vi "Encoder Get To Set Point.vi"(0 "refnum name":string="My Encoder RefNum", 1 "X":dbl, 2 "Y":dbl, 3 "setpoint":dbl format="%.2f", 4 "Enable?":bool) -> (5 "Enable?":bool, 6 "X out":dbl, 7 "Y out":dbl)   [LabVIEW 2016]
doc: "Get to a specific encoder distance (m)."
uses:
  <vilib>/addons/control/pid/pid.llb/PID (DBL).vi
  <vilib>/addons/control/pid/NI_PID_pid.lvlib
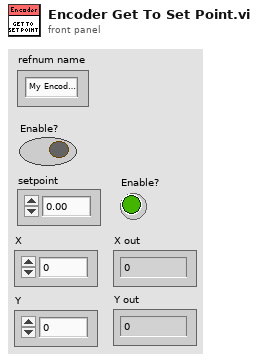
[diagram p1: front panel]
types:
  T1 = cluster{"proportional gain (Kc)":dbl, "integral time (Ti, min)":dbl, "derivative time (Td, min)":dbl}
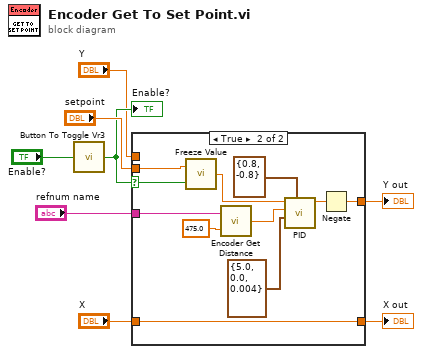
[diagram p0: block diagram]
diagram:
  n1 = call "Button To Toggle Vr3.vi"("InValue"="Enable?") -> ("Result"=w5:bool)
  "Enable?" <- w5
  n2 = case shown="True" w5 {
    selector: w5 -> [_ w12]
    tunnel: "setpoint" -> [_ w14]
    tunnel: "refnum name" -> [_ w18]
    tunnel: [w10 w15] -> w1
    tunnel: [w9 w16] -> w4
    tunnel: "X" -> [w9 w16]
    tunnel: "Y" -> [w10 _]
    frame False {
    }
    frame True {
      n3 = call "Freeze Value.vi"("Freeze Value"=w12, "In Value"=w14) -> ("Value Out"=w13:dbl)
      n4 = call "Encoder Get Distance.vi"("Distance/Meter ratio"=475.0, "refnum name"=w18) -> ("Distance (m)"=w20:dbl)
      n5 = call-poly <vilib>:"PID.vi"("output range"=cluster{"output high":dbl, "output low":dbl} {"output high"=0.8, "output low"=-0.8}, "PID gains"=T1 {"proportional gain (Kc)"=5.0, "integral time (Ti, min)"=0.0, "derivative time (Td, min)"=0.004}, "process variable"=w20, "setpoint"=w13) -> ("output"=w17:dbl)  [unwired: 6 in, 1 out]
      n6 = Negate(x=w17) -> (-x=w15:dbl)
    }
  }
  "X out" <- w4
  "Y out" <- w1
